vi "open.vi"(8 "error in (no error)":errorcluster, 11 "K2602 in":refnum<class "K2602.lvclass">) -> (0 "error out":errorcluster, 3 "K2602 out":refnum<class "K2602.lvclass">)   [LabVIEW 2009, in "Hardware.lvlib" / "Channels.lvlib" / "K2602.lvclass"]
uses:
  K2602.lvclass
  K2602.lvclass/K2602.ctl
  <instrlib>/Keithley 2600 Series/Keithley 2600 Series.lvlib
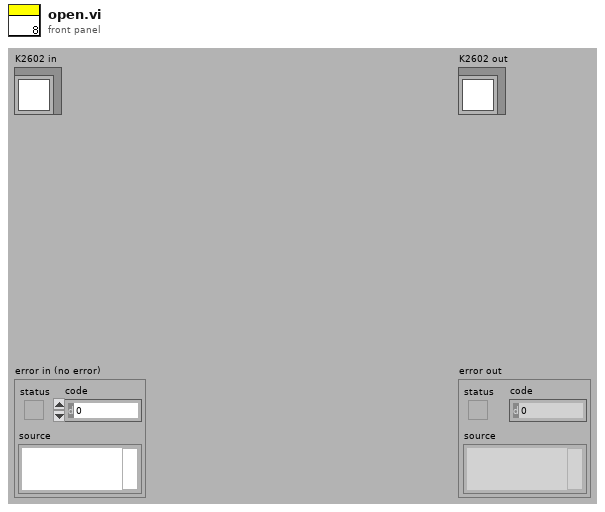
[diagram p1: front panel]
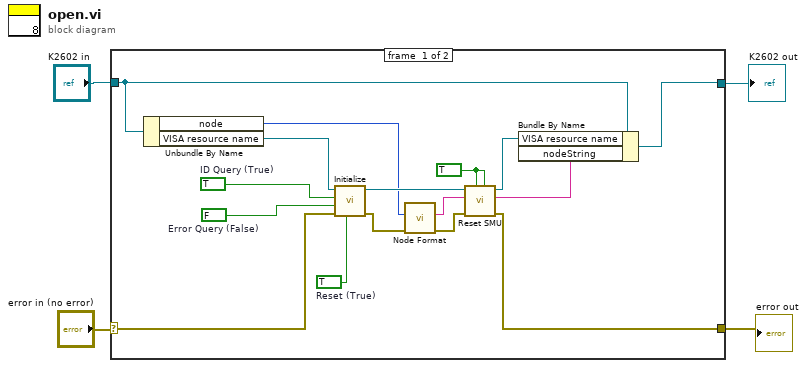
[diagram p0: block diagram]
diagram:
  n1 = case shown="No Error" "error in (no error)" {
    selector: "error in (no error)" -> [w7 w21]
    tunnel: [w10 w22] -> w3
    tunnel: "K2602 in" -> [w11 w22]
    tunnel: [w6 w21] -> w1
    frame #0 {
      w12 = FALSE  # Error Query (False)
      w14 = TRUE
      w18 = TRUE  # Reset (True)
      w20 = TRUE  # ID Query (True)
      n2 = Unbundle By Name(w11) -> ("node"=w13:i8, "VISA resource name"=w5:refnum<visa-resource-name>)
      n3 = call <instrlib>:"Initialize.vi"("Reset (True)"=w18, "error in (no error)"=w7, "Error Query (False)"=w12, "ID Query (True)"=w20, "VISA resource name"=w5) -> ("error out"=w16:errorcluster, "VISA resource name out"=w19:refnum<visa-resource-name>)  [unwired: 1 in, 4 out]
      n4 = call <instrlib>:"Node Format.vi"("error in"=w16, "Node (0-64)"=w13) -> ("error out"=w15:errorcluster, "Formatted Node"=w17:string)  [unwired: 8 out]
      n5 = call <instrlib>:"Reset SMU.vi"("SMU B (No)"=w14, "SMU A (No)"=w14, "error in (no error)"=w15, "Node In"=w17, "VISA resource name"=w19) -> ("error out"=w6:errorcluster, "Node Out"=w8:string, "VISA resource name out"=w9:refnum<visa-resource-name>)  [unwired: 4 out]
      n6 = Bundle By Name(cluster=w11, "VISA resource name"=w9, "nodeString"=w8) -> (w10:refnum<class "K2602.lvclass">)
    }
    frame #1 {
    }
  }
  "error out" <- w1
  "K2602 out" <- w3
